vi "BCU参数读取-Auto.vi"(8 "CAN端口":u16(ring), 9 "设备索引号":u16(ring), 10 "CAN卡类型":u32(ring)=21, 11 "Myindex":dbl=1.0) -> (3 "成功":bool)   [LabVIEW 2013] (continued)
                n4250 = local write "命令序号"(w6047) -> ()
                n4251 = local write "命令"(w6052) -> ()
                n4252 = local write "控制1"(TRUE ("控制1")) -> ()
                n4253 = local write "写?"(FALSE ("写?")) -> ()
                n4254 = local write "消除"(TRUE ("消除")) -> ()
                n4255 = global write "EV05全局变量1.vi" "流控帧 2"(TRUE ("流控帧 2")) -> ()
                n4256 = global write "EV05全局变量1.vi" "流控帧"(FALSE ("流控帧")) -> ()
              }
              frame #2 {
                n4257 = flat-sequence {
                  tunnel: [w6095] -> w6094
                  tunnel: w6094 -> [w6102]
                  frame #0 {
                    n4258 = while {
                      tunnel: [w6096] -> w6095
                      i -> [w6100]
                      stop <- w6097 stop-if-true
                      n4259 = local read "继电器超时处理"() -> (w6096:bool)
                      n4260 = Greater Or Equal?(x=w6100, y=20) -> (x >= y?=w6098:bool)
                      n4261 = Wait Until Next ms Multiple(millisecond multiple=u32 100 ("毫秒倍数")) -> ()  [unwired: 1 out]
                      n4262 = Or(x=w6096, y=w6098) -> (x .or. y?=w6097:bool)
                    }
                  }
                  frame #1 {
                    n4263 = case shown="假" w6102 {
                      frame False {
                        n4264 = local read "DO1"() -> (w6104:bool)
                        n4265 = Not(x=w6104) -> (.not. x?=w6103:bool)
                        n4266 = local write "DO1"(w6103) -> ()
                        n4267 = One Button Dialog(message="DO控制处理超时" ("消息"), button name ("OK")="是" ("按钮名称（“确定”）")) -> ()  [unwired: 1 out]
                      }
                      frame True {
                      }
                    }
                  }
                }
              }
            }
          }
          event "DO2": Value Change {
            n4268 = event-data() -> ("NewVal"=w6107:bool)  [unwired: 6 out]
            n4269 = stacked-sequence {
              tunnel: w6107 -> [_ w6120 _]
              frame #0 {
                w6110 = FALSE ("清BUFF")
                n4270 = local write "继电器超时处理"(FALSE ("继电器超时处理")) -> ()
                n4271 = local write "主从选择"(enum32{"主板", "从板"}."主板" ("主从选择")) -> ()
                n4272 = local write "清BUFF"(w6110) -> ()
                n4273 = local write "正级继电器 10"(w6110) -> ()
              }
              frame #1 {
                n4274 = case shown="真" w6120 {
                  selector: w6120 -> [w6135 w6155]
                  tunnel: [w6134 w6154] -> w6119
                  tunnel: [w6122 w6142] -> w6114
                  frame False {
                    w6130 = 256.0 ("y")
                    w6122 = u32 2 ("命令序号")
                    w6134 = u8 192 ("命令")
                    n4275 = local read "动作保持时间"() -> (w6131:dbl)
                    n4276 = Quotient & Remainder(x=w6131, y=w6130) -> (x-y*floor(x/y)=w6123:dbl, floor(x/y)=w6127:dbl)
                    n4277 = Quotient & Remainder(x=w6127, y=w6130) -> (x-y*floor(x/y)=w6124:dbl, floor(x/y)=w6128:dbl)
                    n4278 = Quotient & Remainder(x=w6128, y=w6130) -> (x-y*floor(x/y)=w6125:dbl, floor(x/y)=w6129:dbl)
                    n4279 = local read "设备索引号"() -> (w6139:u16)
                    n4280 = local read "CAN卡类型"() -> (w6140:u32)
                    n4281 = local read "CAN端口"() -> (w6138:u16)
                    n4282 = Boolean To (0,1)(Boolean=w6135) -> (0, 1=w6132:i16)
                    n4283 = Quotient & Remainder(x=w6129, y=w6130) -> (x-y*floor(x/y)=w6126:dbl)  [unwired: 1 out]
                    n4284 = Build Array(i16 2 ("元素"), w6132, w6126, w6125, w6124, w6123, 0.0 ("元素")) -> (w6136:dbl[])
                    n4285 = call "多帧发送机制(EV05).vi"("can卡类型"=w6140, "设备索引号"=w6139, "CAN端口"=w6138, "命令"=w6134, "板号"=u8 0, "命令序号"=w6122, "输入数据"=w6136) -> ()  [unwired: 2 in, 11 out]
                  }
                  frame True {
                    w6150 = 256.0 ("y")
                    w6142 = u32 2 ("命令序号")
                    w6154 = u8 192 ("命令")
                    n4286 = local read "动作保持时间"() -> (w6151:dbl)
                    n4287 = Quotient & Remainder(x=w6151, y=w6150) -> (x-y*floor(x/y)=w6143:dbl, floor(x/y)=w6147:dbl)
                    n4288 = Quotient & Remainder(x=w6147, y=w6150) -> (x-y*floor(x/y)=w6144:dbl, floor(x/y)=w6148:dbl)
                    n4289 = Quotient & Remainder(x=w6148, y=w6150) -> (x-y*floor(x/y)=w6145:dbl, floor(x/y)=w6149:dbl)
                    n4290 = local read "设备索引号"() -> (w6159:u16)
                    n4291 = local read "CAN卡类型"() -> (w6160:u32)
                    n4292 = local read "CAN端口"() -> (w6158:u16)
                    n4293 = Boolean To (0,1)(Boolean=w6155) -> (0, 1=w6152:i16)
                    n4294 = Quotient & Remainder(x=w6149, y=w6150) -> (x-y*floor(x/y)=w6146:dbl)  [unwired: 1 out]
                    n4295 = Build Array(i16 2 ("元素"), w6152, w6146, w6145, w6144, w6143, 0.0 ("元素")) -> (w6156:dbl[])
                    n4296 = call "多帧发送机制(EV05).vi"("can卡类型"=w6160, "设备索引号"=w6159, "CAN端口"=w6158, "命令"=w6154, "板号"=u8 0, "命令序号"=w6142, "输入数据"=w6156) -> ()  [unwired: 2 in, 11 out]
                  }
                }
                n4297 = local write "命令序号"(w6114) -> ()
                n4298 = local write "命令"(w6119) -> ()
                n4299 = local write "控制1"(TRUE ("控制1")) -> ()
                n4300 = local write "写?"(FALSE ("写?")) -> ()
                n4301 = local write "消除"(TRUE ("消除")) -> ()
                n4302 = global write "EV05全局变量1.vi" "流控帧 2"(TRUE ("流控帧 2")) -> ()
                n4303 = global write "EV05全局变量1.vi" "流控帧"(FALSE ("流控帧")) -> ()
              }
              frame #2 {
                n4304 = flat-sequence {
                  tunnel: [w6162] -> w6161
                  tunnel: w6161 -> [w6169]
                  frame #0 {
                    n4305 = while {
                      tunnel: [w6163] -> w6162
                      i -> [w6167]
                      stop <- w6164 stop-if-true
                      n4306 = local read "继电器超时处理"() -> (w6163:bool)
                      n4307 = Greater Or Equal?(x=w6167, y=20) -> (x >= y?=w6165:bool)
                      n4308 = Wait Until Next ms Multiple(millisecond multiple=u32 100 ("毫秒倍数")) -> ()  [unwired: 1 out]
                      n4309 = Or(x=w6163, y=w6165) -> (x .or. y?=w6164:bool)
                    }
                  }
                  frame #1 {
                    n4310 = case shown="假" w6169 {
                      frame False {
                        n4311 = local read "DO2"() -> (w6171:bool)
                        n4312 = Not(x=w6171) -> (.not. x?=w6170:bool)
                        n4313 = local write "DO2"(w6170) -> ()
                        n4314 = One Button Dialog(message="DO控制处理超时" ("消息"), button name ("OK")="是" ("按钮名称（“确定”）")) -> ()  [unwired: 1 out]
                      }
                      frame True {
                      }
                    }
                  }
                }
              }
            }
          }
          event "DO1 2": Value Change {
            n4315 = event-data() -> ("NewVal"=w6174:bool)  [unwired: 6 out]
            n4316 = stacked-sequence {
              tunnel: w6174 -> [_ w6188 _]
              frame #0 {
                w6177 = FALSE ("继电器超时处理")
                n4317 = local write "继电器超时处理"(w6177) -> ()
                n4318 = local write "正级继电器 11"(w6177) -> ()
                n4319 = local write "主从选择"(enum32{"主板", "从板"}."从板" ("主从选择")) -> ()
              }
              frame #1 {
                n4320 = case shown="假" w6188 {
                  selector: w6188 -> [w6203 w6223]
                  tunnel: [w6202 w6222] -> w6187
                  tunnel: [w6201 w6221] -> w6181
                  tunnel: [w6190 w6210] -> w6182
                  frame True {
                    w6198 = 256.0 ("y")
                    w6190 = u32 2 ("命令序号")
                    w6202 = u8 192 ("命令")
                    n4321 = local read "动作保持时间"() -> (w6199:dbl)
                    n4322 = Quotient & Remainder(x=w6199, y=w6198) -> (x-y*floor(x/y)=w6191:dbl, floor(x/y)=w6195:dbl)
                    n4323 = Quotient & Remainder(x=w6195, y=w6198) -> (x-y*floor(x/y)=w6192:dbl, floor(x/y)=w6196:dbl)
                    n4324 = Quotient & Remainder(x=w6196, y=w6198) -> (x-y*floor(x/y)=w6193:dbl, floor(x/y)=w6197:dbl)
                    n4325 = Quotient & Remainder(x=w6197, y=w6198) -> (x-y*floor(x/y)=w6194:dbl)  [unwired: 1 out]
                    n4326 = Boolean To (0,1)(Boolean=w6203) -> (0, 1=w6200:i16)
                    n4327 = local read "设备索引号"() -> (w6207:u16)
                    n4328 = local read "CAN卡类型"() -> (w6208:u32)
                    n4329 = local read "从板板号"() -> (w6201:u8)
                    n4330 = local read "CAN端口"() -> (w6206:u16)
                    n4331 = Build Array(i16 3 ("元素"), w6200, w6194, w6193, w6192, w6191, 0.0 ("元素")) -> (w6205:dbl[])
                    n4332 = call "多帧发送机制(EV05).vi"("can卡类型"=w6208, "设备索引号"=w6207, "CAN端口"=w6206, "命令"=w6202, "板号"=w6201, "命令序号"=w6190, "输入数据"=w6205) -> ()  [unwired: 2 in, 11 out]
                  }
                  frame False {
                    w6218 = 256.0 ("y")
                    w6210 = u32 2 ("命令序号")
                    w6222 = u8 192 ("命令")
                    n4333 = local read "动作保持时间"() -> (w6219:dbl)
                    n4334 = Quotient & Remainder(x=w6219, y=w6218) -> (x-y*floor(x/y)=w6211:dbl, floor(x/y)=w6215:dbl)
                    n4335 = Quotient & Remainder(x=w6215, y=w6218) -> (x-y*floor(x/y)=w6212:dbl, floor(x/y)=w6216:dbl)
                    n4336 = Quotient & Remainder(x=w6216, y=w6218) -> (x-y*floor(x/y)=w6213:dbl, floor(x/y)=w6217:dbl)
                    n4337 = Quotient & Remainder(x=w6217, y=w6218) -> (x-y*floor(x/y)=w6214:dbl)  [unwired: 1 out]
                    n4338 = Boolean To (0,1)(Boolean=w6223) -> (0, 1=w6220:i16)
                    n4339 = local read "设备索引号"() -> (w6227:u16)
                    n4340 = local read "CAN卡类型"() -> (w6228:u32)
                    n4341 = local read "从板板号"() -> (w6221:u8)
                    n4342 = local read "CAN端口"() -> (w6226:u16)
                    n4343 = Build Array(i16 1 ("元素"), w6220, w6214, w6213, w6212, w6211, 0.0 ("元素")) -> (w6225:dbl[])
                    n4344 = call "多帧发送机制(EV05).vi"("can卡类型"=w6228, "设备索引号"=w6227, "CAN端口"=w6226, "命令"=w6222, "板号"=w6221, "命令序号"=w6210, "输入数据"=w6225) -> ()  [unwired: 2 in, 11 out]
                  }
                }
                n4345 = local write "从板板号"(w6181) -> ()
                n4346 = local write "命令序号"(w6182) -> ()
                n4347 = local write "命令"(w6187) -> ()
                n4348 = local write "清BUFF"(FALSE ("清BUFF")) -> ()
                n4349 = local write "写?"(FALSE ("写?")) -> ()
                n4350 = local write "控制1"(TRUE ("控制1")) -> ()
                n4351 = global write "EV05全局变量1.vi" "流控帧"(FALSE ("流控帧")) -> ()
                n4352 = global write "EV05全局变量1.vi" "流控帧 2"(TRUE ("流控帧 2")) -> ()
                n4353 = local write "消除"(TRUE ("消除")) -> ()
              }
              frame #2 {
                n4354 = flat-sequence {
                  tunnel: [w6230] -> w6229
                  tunnel: w6229 -> [w6237]
                  frame #0 {
                    n4355 = while {
                      tunnel: [w6231] -> w6230
                      i -> [w6235]
                      stop <- w6232 stop-if-true
                      n4356 = local read "继电器超时处理"() -> (w6231:bool)
                      n4357 = Greater Or Equal?(x=w6235, y=20) -> (x >= y?=w6233:bool)
                      n4358 = Wait Until Next ms Multiple(millisecond multiple=u32 100 ("毫秒倍数")) -> ()  [unwired: 1 out]
                      n4359 = Or(x=w6231, y=w6233) -> (x .or. y?=w6232:bool)
                    }
                  }
                  frame #1 {
                    n4360 = case shown="假" w6237 {
                      frame False {
                        n4361 = local read "DO1 2"() -> (w6239:bool)
                        n4362 = Not(x=w6239) -> (.not. x?=w6238:bool)
                        n4363 = local write "DO1 2"(w6238) -> ()
                        n4364 = One Button Dialog(message="DO控制处理超时" ("消息"), button name ("OK")="是" ("按钮名称（“确定”）")) -> ()  [unwired: 1 out]
                      }
                      frame True {
                      }
                    }
                  }
                }
              }
            }
          }
          event "读取转换为写入": Value Change {
            n4365 = event-data() -> ("NewVal"=w6242:bool)  [unwired: 6 out]
            n4366 = case shown="真" w6242 {
              tunnel: w6246 -> [w6248 w6253]
              tunnel: [w6248 w6252] -> w6245
              tunnel: w6244 -> [w6247 w6251]
              tunnel: [w6247 w6250] -> w6243
              frame False {
              }
              frame True {
                n4367 = Enqueue Element(queue=w6253, element="读取转换为写入", error in (no error)=w6251) -> (queue out=w6252:refnum<queue>, error out=w6250:errorcluster)  [unwired: 2 out]
              }
            }
          }
          event "读取故障详细状态": Value Change {
            n4368 = event-data() -> ("NewVal"=w6258:bool)  [unwired: 5 out]
            n4369 = case shown="真" w6258 {
              tunnel: w6257 -> [w6260 w6273]
              tunnel: w6256 -> [w6259 w6272]
              tunnel: [w6260 w6271] -> w6255
              tunnel: [w6259 w6270] -> w6254
              frame False {
              }
              frame True {
                n4370 = disable-structure shown="启用" {
                  disable-tunnel: [w6282 TRUE ("发送成功")] -> w6269
                  frame Disabled {
                    n4371 = local read "主从选择"() -> (w6274:enum32{"主板", "从板"})
                    n4372 = case shown="\"主板\", 默认" w6274 {
                      tunnel: [0.0 ("FUNC") w6284] -> w6279
                      frame "主板", Default {
                      }
                      frame "从板" {
                        n4373 = local read "从板号"() -> (w6284:u8)
                      }
                    }
                    n4374 = local read "设备索引号"() -> (w6276:u16)
                    n4375 = local read "CAN卡类型"() -> (w6277:u32)
                    n4376 = local read "CAN端口"() -> (w6275:u16)
                    n4377 = call "标定授权发送.vi"("CAN卡类型"=w6277, "解锁类型"=enum16{"读取", "写", "下载"}."写", "设备索引号"=w6276, "CAN端口"=w6275, "是否连接"=TRUE, "板选择"=0, "FUNC"=w6279) -> ("发送成功"=w6282:bool)  [unwired: 8 out]
                  }
                  frame Enabled {
                  }
                }
                n4378 = case shown="真" w6269 {
                  tunnel: w6273 -> [w6287 w6292]
                  tunnel: w6272 -> [w6286 w6291]
                  tunnel: [w6287 w6289] -> w6271
                  tunnel: [w6286 w6288] -> w6270
                  frame False {
                  }
                  frame True {
                    n4379 = Enqueue Element(queue=w6292, element="读取故障状态" ("元素"), error in (no error)=w6291) -> (queue out=w6289:refnum<queue>, error out=w6288:errorcluster)  [unwired: 2 out]
                  }
                }
                n4380 = local write "电池故障"(string[][] []) -> ()
                n4381 = global write "EV05全局变量1.vi" "流控帧 2"(TRUE ("流控帧")) -> ()
                n4382 = local write "写?"(FALSE ("写?")) -> ()
                n4383 = local write "控制1"(TRUE ("控制1")) -> ()
                n4384 = local write "消除"(TRUE ("消除")) -> ()
                n4385 = local write "清BUFF"(FALSE ("清BUFF")) -> ()
                n4386 = global write "EV05全局变量1.vi" "流控帧"(FALSE ("流控帧")) -> ()
                n4387 = call <vilib>:"Set Busy.vi"("disable click? (T)"=FALSE) -> ()  [unwired: 3 in, 8 out]
              }
            }
          }
          event "项目软本读取": Value Change {
            n4388 = event-data() -> ("NewVal"=w6297:bool)  [unwired: 5 out]
            n4389 = case shown="真" w6297 {
              tunnel: w6296 -> [w6299 w6304]
              tunnel: w6295 -> [w6298 w6303]
              tunnel: [w6299 w6302] -> w6294
              tunnel: [w6298 w6301] -> w6293
              frame False {
              }
              frame True {
                n4390 = stacked-sequence {
                  tunnel: [w6307] -> _
                  frame #0 {
                    w6307 = FALSE ("disable click? (T)")
                    w6310 = FALSE ("写?")
                    n4391 = local write "写?"(w6310) -> ()
                    n4392 = global write "EV05全局变量1.vi" "写入超时"(w6310) -> ()
                    n4393 = local write "项目软件版本号"(" " ("项目软件版本号")) -> ()
                    n4394 = global write "EV05全局变量1.vi" "流控帧"(FALSE ("流控帧")) -> ()
                    n4395 = local write "主从选择"(enum32{"主板", "从板"}."主板" ("主从选择")) -> ()
                    n4396 = call <vilib>:"Set Busy.vi"("disable click? (T)"=w6307) -> ()  [unwired: 3 in, 8 out]
                    n4397 = local write "清BUFF"(FALSE ("清BUFF")) -> ()
                    n4398 = property on="保存版本信息" class="Bool (严格)"("Visible"=TRUE ("可见")) -> ()  [unwired: 2 in, 2 out]
                    n4399 = global write "EV05全局变量1.vi" "流控帧 2"(TRUE ("流控帧 2")) -> ()
                    n4400 = local write "控制1"(TRUE ("控制1")) -> ()
                    n4401 = local write "消除"(TRUE ("消除")) -> ()
                  }
                }
                n4402 = Enqueue Element(queue=w6304, element="项目软件版本读取" ("元素"), error in (no error)=w6303) -> (queue out=w6302:refnum<queue>, error out=w6301:errorcluster)  [unwired: 2 out]
              }
            }
          }
          event "读硬件版本号": Value Change {
            n4403 = event-data() -> ("NewVal"=w6319:bool)  [unwired: 5 out]
            n4404 = case shown="真" w6319 {
              tunnel: w6318 -> [w6321 w6328]
              tunnel: w6317 -> [w6320 w6327]
              tunnel: [w6321 w6326] -> w6316
              tunnel: [w6320 w6325] -> w6315
              frame False {
              }
              frame True {
                n4405 = global read "EV05全局变量1.vi" "授权功能"() -> (w6323:bool)
                n4406 = case shown="真" w6323 {
                  tunnel: [TRUE ("发送成功") w6347] -> w6324
                  frame False {
                  }
                  frame True {
                    n4407 = local read "设备索引号"() -> (w6342:u16)
                    n4408 = local read "CAN卡类型"() -> (w6343:u32)
                    n4409 = local read "CAN端口"() -> (w6341:u16)
                    n4410 = call "标定授权发送.vi"("CAN卡类型"=w6343, "解锁类型"=enum16{"读取", "写", "下载"}."读取", "设备索引号"=w6342, "CAN端口"=w6341, "是否连接"=TRUE, "板选择"=0, "FUNC"=u32 0) -> ("发送成功"=w6347:bool)  [unwired: 8 in]
                  }
                }
                n4411 = stacked-sequence {
                  tunnel: [w6331] -> w6322
                  frame #0 {
                    w6331 = TRUE ("控制1")
                    w6335 = FALSE ("写?")
                    n4412 = local write "写?"(w6335) -> ()
                    n4413 = global write "EV05全局变量1.vi" "写入超时"(w6335) -> ()
                    n4414 = call <vilib>:"Set Busy.vi"("disable click? (T)"=FALSE) -> ()  [unwired: 3 in, 8 out]
                    n4415 = local write "硬件版本号"("" ("硬件版本号")) -> ()
                    n4416 = property on="保存版本信息" class="Bool (严格)"("Visible"=TRUE ("可见")) -> ()  [unwired: 2 in, 2 out]
                    n4417 = local write "主从选择"(enum32{"主板", "从板"}."主板" ("主从选择")) -> ()
                    n4418 = local write "控制1"(w6331) -> ()
                    n4419 = local write "清BUFF"(FALSE ("清BUFF")) -> ()
                    n4420 = global write "EV05全局变量1.vi" "流控帧 2"(TRUE ("流控帧 2")) -> ()
                    n4421 = local write "消除"(TRUE ("消除")) -> ()
                    n4422 = global write "EV05全局变量1.vi" "流控帧"(FALSE ("流控帧")) -> ()
                  }
                }
                n4423 = case shown="真" w6324 {
                  tunnel: w6328 -> [w6349 w6354]
                  tunnel: w6327 -> [w6348 w6353]
                  tunnel: [w6349 w6351] -> w6326
                  tunnel: [w6348 w6350] -> w6325
                  tunnel: w6322 -> [_ _]
                  frame False {
                  }
                  frame True {
                    n4424 = Enqueue Element(queue=w6354, element="硬件版本读取" ("元素"), error in (no error)=w6353) -> (queue out=w6351:refnum<queue>, error out=w6350:errorcluster)  [unwired: 2 out]
                  }
                }
              }
            }
          }
          event "平台软件版本读取": Value Change {
            n4425 = event-data() -> ("NewVal"=w6359:bool)  [unwired: 5 out]
            n4426 = case shown="真" w6359 {
              tunnel: w6358 -> [w6361 w6366]
              tunnel: w6357 -> [w6360 w6365]
              tunnel: [w6361 w6364] -> w6356
              tunnel: [w6360 w6363] -> w6355
              frame False {
              }
              frame True {
                n4427 = stacked-sequence {
                  tunnel: [w6369] -> _
                  frame #0 {
                    w6369 = TRUE ("控制1")
                    w6373 = FALSE ("写?")
                    n4428 = call <vilib>:"Set Busy.vi"("disable click? (T)"=FALSE) -> ()  [unwired: 3 in, 8 out]
                    n4429 = local write "写?"(w6373) -> ()
                    n4430 = global write "EV05全局变量1.vi" "写入超时"(w6373) -> ()
                    n4431 = local write "平台软件版本号"(" " ("平台软件版本号")) -> ()
                    n4432 = local write "控制1"(w6369) -> ()
                    n4433 = local write "消除"(TRUE ("消除")) -> ()
                    n4434 = property on="保存版本信息" class="Bool (严格)"("Visible"=TRUE ("可见")) -> ()  [unwired: 2 in, 2 out]
                    n4435 = global write "EV05全局变量1.vi" "流控帧 2"(TRUE ("流控帧 2")) -> ()
                    n4436 = local write "主从选择"(enum32{"主板", "从板"}."主板" ("主从选择")) -> ()
                    n4437 = local write "清BUFF"(FALSE ("清BUFF")) -> ()
                    n4438 = global write "EV05全局变量1.vi" "流控帧"(FALSE ("流控帧")) -> ()
                  }
                }
                n4439 = Enqueue Element(queue=w6366, element="平台软件版本读取" ("元素"), error in (no error)=w6365) -> (queue out=w6364:refnum<queue>, error out=w6363:errorcluster)  [unwired: 2 out]
              }
            }
          }
          event "模块版本读取": Value Change {
            n4440 = event-data() -> ("NewVal"=w6381:bool)  [unwired: 5 out]
            n4441 = case shown="真" w6381 {
              tunnel: w6380 -> [w6383 w6390]
              tunnel: w6379 -> [w6382 w6389]
              tunnel: [w6383 w6388] -> w6378
              tunnel: [w6382 w6387] -> w6377
              frame False {
              }
              frame True {
                n4442 = global read "EV05全局变量1.vi" "授权功能"() -> (w6385:bool)
                n4443 = case shown="假" w6385 {
                  tunnel: [TRUE ("发送成功") w6408] -> w6386
                  frame False {
                  }
                  frame True {
                    n4444 = local read "设备索引号"() -> (w6403:u16)
                    n4445 = local read "CAN卡类型"() -> (w6404:u32)
                    n4446 = local read "CAN端口"() -> (w6402:u16)
                    n4447 = call "标定授权发送.vi"("CAN卡类型"=w6404, "解锁类型"=enum16{"读取", "写", "下载"}."读取", "设备索引号"=w6403, "CAN端口"=w6402, "是否连接"=TRUE, "板选择"=0, "FUNC"=u32 0) -> ("发送成功"=w6408:bool)  [unwired: 8 out]
                  }
                }
                n4448 = stacked-sequence {
                  tunnel: [w6393] -> w6384
                  frame #0 {
                    w6393 = TRUE ("控制1")
                    w6396 = FALSE ("写?")
                    n4449 = call <vilib>:"Set Busy.vi"("disable click? (T)"=FALSE) -> ()  [unwired: 3 in, 8 out]
                    n4450 = local write "写?"(w6396) -> ()
                    n4451 = global write "EV05全局变量1.vi" "写入超时"(w6396) -> ()
                    n4452 = local write "主从选择"(enum32{"主板", "从板"}."主板" ("主从选择")) -> ()
                    n4453 = local write "清BUFF"(FALSE ("清BUFF")) -> ()
                    n4454 = property on="保存版本信息" class="Bool (严格)"("Visible"=TRUE ("可见")) -> ()  [unwired: 2 in, 2 out]
                    n4455 = global write "EV05全局变量1.vi" "流控帧 2"(TRUE ("流控帧 2")) -> ()
                    n4456 = local write "控制1"(w6393) -> ()
                    n4457 = local write "消除"(TRUE ("消除")) -> ()
                    n4458 = global write "EV05全局变量1.vi" "流控帧"(FALSE ("流控帧")) -> ()
                  }
                }
                n4459 = case shown="真" w6386 {
                  tunnel: w6390 -> [w6410 w6415]
                  tunnel: w6389 -> [w6409 w6414]
                  tunnel: [w6410 w6412] -> w6388
                  tunnel: [w6409 w6411] -> w6387
                  tunnel: w6384 -> [_ _]
                  frame False {
                  }
                  frame True {
                    n4460 = Enqueue Element(queue=w6415, element="模块软件版本读取" ("元素"), error in (no error)=w6414) -> (queue out=w6412:refnum<queue>, error out=w6411:errorcluster)  [unwired: 2 out]
                  }
                }
              }
            }
          }
          event "保存版本信息": Value Change {
            n4461 = event-data() -> ("NewVal"=w6416:bool)  [unwired: 6 out]
            n4462 = case shown="真" w6416 {
              frame False {
              }
              frame True {
                n4463 = stacked-sequence {
                  seq-local: [w6420 _] -> [_ w6422]
                  seq-local: [w6419 _] -> [_ w6421]
                  frame #0 {
                    n4464 = call "请输入从板个数"() -> ("从板个数"=w6420:dbl, "确定"=w6419:bool)  [unwired: 17 in, 1 out]
                  }
                  frame #1 {
                    n4465 = case shown="真" w6421 {
                      tunnel: w6422 -> [_ w6425]
                      frame False {
                      }
                      frame True {
                        n4466 = call <vilib>:"Application Directory.vi"() -> ("Application Directory"=w6437:path)
                        n4467 = Build Path(base path=w6437, name or relative path="SaveData" ("名称或相对路径")) -> (appended path=w6435:path)
                        n4468 = local read "模块版本名称"() -> (w6430:string[][])
                        n4469 = local read "项目软件版本"() -> (w6427:string[])
                        n4470 = local read "模块版本值"() -> (w6429:string[][])
                        n4471 = local read "平台软件版本"() -> (w6426:string[])
                        n4472 = local read "模块个数"() -> (w6423:u8[])
                        n4473 = local read "硬件版本"() -> (w6428:string[])
                        n4474 = call "文件对话框3"("start path"=w6435, "prompt"="选择要保存数据的位置", "default name"="BMS版本信息.txt") -> ("selected path"=w6431:path, "cancelled"=w6432:bool)  [unwired: 9 in, 2 out]
                        n4475 = Increment(x=w6425) -> (x+1=w6424:dbl)
                        n4476 = for {
                          N: w6424 -> [_]
                          tunnel: w6432 -> [w6453]
                          tunnel: w6431 -> [w6452]
                          tunnel: w6430 -> [w6442] mode=indexing
                          tunnel: w6429 -> [w6440] mode=indexing
                          tunnel: w6428 -> [w6447] mode=indexing
                          tunnel: w6427 -> [w6446] mode=indexing
                          tunnel: w6426 -> [w6445] mode=indexing
                          tunnel: w6423 -> [w6438] mode=indexing
                          i -> [w6444]
                          w6450 = ""
                          w6457 = 0 ("索引")
                          n4477 = case shown="0, 默认" w6444 {
                            selector: w6444 -> [_ w6471]
                            tunnel: ["主板版本信息" w6472] -> w6462
                            tunnel: [FALSE TRUE] -> w6448
                            frame 0, Default {
                            }
                            frame 1.. {
                              n4478 = Number To Decimal String(number=w6471) -> (decimal integer string=w6470:string)  [unwired: 1 in]
                              n4479 = Concatenate Strings("从板", w6470, "版本信息") -> (w6472:string)
                            }
                          }
                          n4480 = Increment(x=w6438) -> (x+1=w6439:u8)
                          n4481 = Array Subset(array=w6442, length=w6439) -> (w6443:string[])  [unwired: 1 in]
                          n4482 = Array Subset(array=w6440, length=w6439) -> (w6441:string[])  [unwired: 1 in]
                          n4483 = Build Array(w6450, w6445, w6446, w6447, w6450) -> (w6456:string[])
                          n4484 = Build Array(w6462, "平台软件版本号", "项目软件版本号", "硬件版本号", "模块版本号") -> (w6458:string[])
                          n4485 = Insert Into Array(array=w6443, index=w6457, new element=w6458) -> (w6455:string[])
                          n4486 = Insert Into Array(array=w6441, index=w6457, new element=w6456) -> (w6454:string[])
                          n4487 = Build Array(w6455, w6454) -> (w6451:string[][])
                          n4488 = case shown="假" w6453 {
                            tunnel: w6452 -> [w6466 _]
                            tunnel: w6451 -> [w6465 _]
                            tunnel: w6448 -> [w6463 _]
                            frame False {
                              n4489 = call-poly <vilib>:"Write To Spreadsheet File.vi"("transpose? (no:F)"=TRUE, "append to file? (new file:F)"=w6463, "2D data"=w6465, "file path (dialog if empty)"=w6466) -> ()  [unwired: 4 in, 1 out]
                            }
                            frame True {
                            }
                          }
                        }
                      }
                    }
                  }
                }
              }
            }
          }
          event "单个写入": Value Change {
            n4490 = event-data() -> ("NewVal"=w6479:bool)  [unwired: 5 out]
            n4491 = case shown="真" w6479 {
              tunnel: w6478 -> [w6481 w6488]
              tunnel: w6477 -> [w6480 w6487]
              tunnel: [w6481 w6486] -> w6476
              tunnel: [w6480 w6485] -> w6475
              frame False {
              }
              frame True {
                w6483 = FALSE ("流控帧")
                w6482 = TRUE ("流控帧 2")
                n4492 = disable-structure shown="禁用" {
                  disable-tunnel: [w6497 TRUE ("发送成功")] -> w6484
                  frame Disabled {
                    n4493 = local read "主从选择"() -> (w6489:enum32{"主板", "从板"})
                    n4494 = case shown="\"主板\", 默认" w6489 {
                      tunnel: [0.0 ("FUNC") w6499] -> w6494
                      frame "主板", Default {
                      }
                      frame "从板" {
                        n4495 = local read "从板号"() -> (w6499:u8)
                      }
                    }
                    n4496 = local read "设备索引号"() -> (w6491:u16)
                    n4497 = local read "CAN卡类型"() -> (w6492:u32)
                    n4498 = local read "CAN端口"() -> (w6490:u16)
                    n4499 = call "标定授权发送.vi"("CAN卡类型"=w6492, "解锁类型"=enum16{"读取", "写", "下载"}."写", "设备索引号"=w6491, "CAN端口"=w6490, "是否连接"=TRUE, "板选择"=0, "FUNC"=w6494) -> ("发送成功"=w6497:bool)  [unwired: 8 out]
                  }
                  frame Enabled {
                  }
                }
                n4500 = case shown="真" w6484 {
                  tunnel: w6488 -> [w6502 w6506]
                  tunnel: w6487 -> [w6501 w6505]
                  tunnel: [w6502 w6508] -> w6486
                  tunnel: [w6501 w6507] -> w6485
                  frame False {
                  }
                  frame True {
                    n4501 = Flush Queue(queue=w6506, error in (no error)=w6505) -> (queue out=w6504:refnum<queue>, error out=w6503:errorcluster)  [unwired: 1 out]
                    n4502 = Enqueue Element(queue=w6504, element="单个写入" ("元素"), error in (no error)=w6503) -> (queue out=w6508:refnum<queue>, error out=w6507:errorcluster)  [unwired: 2 out]
                  }
                }
                n4503 = global write "EV05全局变量1.vi" "读取超时"(w6483) -> ()
                n4504 = global write "EV05全局变量1.vi" "流控帧"(w6483) -> ()
                n4505 = local write "消除"(w6482) -> ()
                n4506 = local write "控制1"(w6482) -> ()
                n4507 = global write "EV05全局变量1.vi" "流控帧 2"(w6482) -> ()
                n4508 = local write "写?"(w6482) -> ()
              }
            }
          }
          event "全部写入": Value Change {
            n4509 = event-data() -> ("NewVal"=w6514:bool)  [unwired: 5 out]
            n4510 = case shown="真" w6514 {
              tunnel: w6513 -> [w6516 w6524]
              tunnel: w6512 -> [w6515 w6523]
              tunnel: [w6516 w6522] -> w6511
              tunnel: [w6515 w6521] -> w6510
              frame False {
              }
              frame True {
                w6518 = FALSE ("流控帧")
                w6517 = TRUE ("流控帧 2")
                n4511 = global read "EV05全局变量1.vi" "授权功能"() -> (w6519:bool)
                n4512 = case shown="真" w6519 {
                  tunnel: [TRUE ("发送成功") w6534] -> w6520
                  frame False {
                  }
                  frame True {
                    n4513 = local read "主从选择"() -> (w6526:enum32{"主板", "从板"})
                    n4514 = case shown="\"从板\"" w6526 {
                      tunnel: [0.0 ("FUNC") w6536] -> w6527
                      frame "主板", Default {
                      }
                      frame "从板" {
                        n4515 = local read "从板号"() -> (w6536:u8)
                      }
                    }
                    n4516 = local read "设备索引号"() -> (w6529:u16)
                    n4517 = local read "CAN卡类型"() -> (w6530:u32)
                    n4518 = local read "CAN端口"() -> (w6528:u16)
                    n4519 = call "标定授权发送.vi"("CAN卡类型"=w6530, "解锁类型"=enum16{"读取", "写", "下载"}."写", "设备索引号"=w6529, "CAN端口"=w6528, "是否连接"=TRUE, "板选择"=0, "FUNC"=w6527) -> ("发送成功"=w6534:bool)  [unwired: 8 out]
                  }
                }
                n4520 = case shown="真" w6520 {
                  tunnel: w6524 -> [w6538 w6542]
                  tunnel: w6523 -> [w6537 w6541]
                  tunnel: [w6538 w6544] -> w6522
                  tunnel: [w6537 w6543] -> w6521
                  frame False {
                  }
                  frame True {
                    n4521 = Flush Queue(queue=w6542, error in (no error)=w6541) -> (queue out=w6540:refnum<queue>, error out=w6539:errorcluster)  [unwired: 1 out]
                    n4522 = Enqueue Element(queue=w6540, element="全部写入" ("元素"), error in (no error)=w6539) -> (queue out=w6544:refnum<queue>, error out=w6543:errorcluster)  [unwired: 1 in, 1 out]
                  }
                }
                n4523 = global write "EV05全局变量1.vi" "读取超时"(w6518) -> ()
                n4524 = global write "EV05全局变量1.vi" "流控帧"(w6518) -> ()
                n4525 = local write "消除"(w6517) -> ()
                n4526 = local write "控制1"(w6517) -> ()
                n4527 = global write "EV05全局变量1.vi" "流控帧 2"(w6517) -> ()
                n4528 = local write "写?"(w6517) -> ()
              }
            }
          }
          event "单个读取": Value Change {
            n4529 = event-data() -> ("NewVal"=w6550:bool)  [unwired: 5 out]
            n4530 = case shown="真" w6550 {
              tunnel: w6549 -> [w6552 w6560]
              tunnel: w6548 -> [w6551 w6559]
              tunnel: [w6552 w6558] -> w6547
              tunnel: [w6551 w6557] -> w6546
              frame False {
              }
              frame True {
                w6553 = FALSE ("流控帧")
                w6554 = TRUE ("流控帧 2")
                n4531 = global read "EV05全局变量1.vi" "授权功能"() -> (w6555:bool)
                n4532 = case shown="假" w6555 {
                  tunnel: [TRUE ("发送成功") w6569] -> w6556
                  frame False {
                  }
                  frame True {
                    n4533 = local read "设备索引号"() -> (w6563:u16)
                    n4534 = local read "CAN卡类型"() -> (w6564:u32)
                    n4535 = local read "CAN端口"() -> (w6562:u16)
                    n4536 = call "标定授权发送.vi"("CAN卡类型"=w6564, "解锁类型"=enum16{"读取", "写", "下载"}."读取", "设备索引号"=w6563, "CAN端口"=w6562, "是否连接"=TRUE, "板选择"=0, "FUNC"=u32 1) -> ("发送成功"=w6569:bool)  [unwired: 8 out]
                  }
                }
                n4537 = case shown="真" w6556 {
                  tunnel: w6560 -> [w6571 w6575]
                  tunnel: w6559 -> [w6570 w6573]
                  tunnel: [w6571 w6577] -> w6558
                  tunnel: [w6570 w6576] -> w6557
                  frame False {
                  }
                  frame True {
                    n4538 = Flush Queue(queue=w6575, error in (no error)=w6573) -> (queue out=w6574:refnum<queue>, error out=w6572:errorcluster)  [unwired: 1 out]
                    n4539 = Enqueue Element(queue=w6574, element="单个读取" ("元素"), error in (no error)=w6572) -> (queue out=w6577:refnum<queue>, error out=w6576:errorcluster)  [unwired: 2 out]
                  }
                }
                n4540 = global write "EV05全局变量1.vi" "写入超时"(w6553) -> ()
                n4541 = global write "EV05全局变量1.vi" "流控帧"(w6553) -> ()
                n4542 = local write "写?"(w6553) -> ()
                n4543 = local write "消除"(w6554) -> ()
                n4544 = local write "控制1"(w6554) -> ()
                n4545 = global write "EV05全局变量1.vi" "流控帧 2"(w6554) -> ()
              }
            }
          }
          event "全部读取": Value Change {
            n4546 = event-data() -> ("NewVal"=w6583:bool)  [unwired: 5 out]
            n4547 = case shown="真" w6583 {
              tunnel: w6582 -> [w6585 w6589]
              tunnel: w6581 -> [w6584 w6588]
              tunnel: [w6585 w6587] -> w6580
              tunnel: [w6584 w6586] -> w6579
              frame False {
              }
              frame True {
                n4548 = stacked-sequence {
                  seq-local: [w6594 _] -> [_ _]
                  seq-local: [w6593 _] -> [_ _]
                  tunnel: w6589 -> [w6596 w6625]
                  tunnel: w6588 -> [w6595 w6624]
                  tunnel: [_ w6629] -> w6587
                  tunnel: [_ w6628] -> w6586
                  frame #0 {
                    w6590 = FALSE ("布尔")
                    n4549 = local read "路径"() -> (w6592:path)
                    n4550 = Empty String/Path?(string/path=w6592) -> (empty?=w6591:bool)
                    n4551 = case shown="假" w6591 {
                      tunnel: w6596 -> [w6603 w6621]
                      tunnel: w6595 -> [w6602 w6620]
                      tunnel: [w6599 w6620] -> w6594
                      tunnel: [w6598 w6621] -> w6593
                      frame False {
                        n4552 = global read "EV05全局变量1.vi" "授权功能"() -> (w6600:bool)
                        n4553 = case shown="真" w6600 {
                          tunnel: [TRUE ("发送成功") w6612] -> w6601
                          frame False {
                          }
                          frame True {
                            n4554 = local read "设备索引号"() -> (w6606:u16)
                            n4555 = local read "CAN卡类型"() -> (w6607:u32)
                            n4556 = local read "CAN端口"() -> (w6605:u16)
                            n4557 = call "标定授权发送.vi"("CAN卡类型"=w6607, "解锁类型"=enum16{"读取", "写", "下载"}."读取", "设备索引号"=w6606, "CAN端口"=w6605, "是否连接"=TRUE, "板选择"=0, "FUNC"=u32 1) -> ("发送成功"=w6612:bool)  [unwired: 8 out]
                          }
                        }
                        n4558 = case shown="真" w6601 {
                          tunnel: w6603 -> [w6614 w6619]
                          tunnel: w6602 -> [w6613 w6618]
                          tunnel: [w6614 w6616] -> w6598
                          tunnel: [w6613 w6615] -> w6599
                          frame False {
                          }
                          frame True {
                            n4559 = Enqueue Element(queue=w6619, element="读配置文件" ("元素"), error in (no error)=w6618) -> (queue out=w6616:refnum<queue>, error out=w6615:errorcluster)  [unwired: 2 out]
                          }
                        }
                        n4560 = Wait Until Next ms Multiple(millisecond multiple=u32 200 ("毫秒倍数")) -> ()  [unwired: 1 out]
                      }
                      frame True {
                      }
                    }
                    n4561 = local write "1 6"(w6590) -> ()
                    n4562 = local write "1 7"(w6590) -> ()
                    n4563 = local write "1 8"(w6590) -> ()
                    n4564 = local write "1 9"(w6590) -> ()
                    n4565 = local write "1 10"(w6590) -> ()
                    n4566 = local write "1 12"(w6590) -> ()
                  }
                  frame #1 {
                    w6622 = FALSE ("流控帧")
                    w6623 = TRUE ("流控帧 2")
                    n4567 = global read "EV05全局变量1.vi" "授权功能"() -> (w6626:bool)
                    n4568 = case shown="假" w6626 {
                      tunnel: [TRUE ("发送成功") w6638] -> w6627
                      frame False {
                      }
                      frame True {
                        n4569 = local read "设备索引号"() -> (w6632:u16)
                        n4570 = local read "CAN卡类型"() -> (w6633:u32)
                        n4571 = local read "CAN端口"() -> (w6631:u16)
                        n4572 = call "标定授权发送.vi"("CAN卡类型"=w6633, "解锁类型"=enum16{"读取", "写", "下载"}."读取", "设备索引号"=w6632, "CAN端口"=w6631, "是否连接"=TRUE, "板选择"=0, "FUNC"=u32 1) -> ("发送成功"=w6638:bool)  [unwired: 8 out]
                      }
                    }
                    n4573 = case shown="真" w6627 {
                      tunnel: w6625 -> [w6640 w6641]
                      tunnel: w6624 -> [w6639 w6644]
                      tunnel: [w6640 w6646] -> w6629
                      tunnel: [w6639 w6645] -> w6628
                      frame False {
                      }
                      frame True {
                        n4574 = Flush Queue(queue=w6641, error in (no error)=w6644) -> (queue out=w6642:refnum<queue>, error out=w6643:errorcluster)  [unwired: 1 out]
                        n4575 = Enqueue Element(queue=w6642, element="全部读取" ("元素"), error in (no error)=w6643) -> (queue out=w6646:refnum<queue>, error out=w6645:errorcluster)  [unwired: 2 out]
                      }
                    }
                    n4576 = global write "EV05全局变量1.vi" "写入超时"(w6622) -> ()
                    n4577 = global write "EV05全局变量1.vi" "流控帧"(w6622) -> ()
                    n4578 = local write "写?"(w6622) -> ()
                    n4579 = local write "消除"(w6623) -> ()
                    n4580 = local write "控制1"(w6623) -> ()
                    n4581 = global write "EV05全局变量1.vi" "流控帧 2"(w6623) -> ()
                  }
                }
              }
            }
          }
          event "开启均衡": Value Change {
            n4582 = event-data() -> ("NewVal"=w6652:bool)  [unwired: 5 out]
            n4583 = case shown="真" w6652 {
              tunnel: w6651 -> [w6654 w6661]
              tunnel: w6650 -> [w6653 w6660]
              tunnel: [w6654 w6659] -> w6649
              tunnel: [w6653 w6658] -> w6648
              frame False {
              }
              frame True {
                n4584 = global read "EV05全局变量1.vi" "授权功能"() -> (w6656:bool)
                n4585 = case shown="假" w6656 {
                  tunnel: [TRUE ("发送成功") w6671] -> w6657
                  frame False {
                  }
                  frame True {
                    n4586 = local read "主从选择"() -> (w6663:enum32{"主板", "从板"})
                    n4587 = case shown="\"从板\"" w6663 {
                      tunnel: [0.0 ("FUNC") w6673] -> w6664
                      frame "主板", Default {
                      }
                      frame "从板" {
                        n4588 = local read "从板号"() -> (w6673:u8)
                      }
                    }
                    n4589 = local read "设备索引号"() -> (w6666:u16)
                    n4590 = local read "CAN卡类型"() -> (w6667:u32)
                    n4591 = local read "CAN端口"() -> (w6665:u16)
                    n4592 = call "标定授权发送.vi"("CAN卡类型"=w6667, "解锁类型"=enum16{"读取", "写", "下载"}."写", "设备索引号"=w6666, "CAN端口"=w6665, "是否连接"=TRUE, "板选择"=0, "FUNC"=w6664) -> ("发送成功"=w6671:bool)  [unwired: 8 out]
                  }
                }
                n4593 = case shown="真" w6657 {
                  tunnel: w6661 -> [w6675 w6680]
                  tunnel: w6660 -> [w6674 w6679]
                  tunnel: [w6675 w6677] -> w6659
                  tunnel: [w6674 w6676] -> w6658
                  frame False {
                  }
                  frame True {
                    n4594 = Enqueue Element(queue=w6680, element="开启均衡" ("元素"), error in (no error)=w6679) -> (queue out=w6677:refnum<queue>, error out=w6676:errorcluster)  [unwired: 2 out]
                  }
                }
                n4595 = call <vilib>:"Set Busy.vi"("disable click? (T)"=TRUE) -> ()  [unwired: 3 in, 8 out]
              }
            }
          }
          event "关闭均衡": Value Change {
            n4596 = event-data() -> ("NewVal"=w6685:bool)  [unwired: 5 out]
            n4597 = case shown="真" w6685 {
              tunnel: w6684 -> [w6687 w6694]
              tunnel: w6683 -> [w6686 w6693]
              tunnel: [w6687 w6692] -> w6682
              tunnel: [w6686 w6691] -> w6681
              frame False {
              }
              frame True {
                n4598 = global read "EV05全局变量1.vi" "授权功能"() -> (w6689:bool)
                n4599 = case shown="假" w6689 {
                  tunnel: [TRUE ("发送成功") w6704] -> w6690
                  frame False {
                  }
                  frame True {
                    n4600 = local read "主从选择"() -> (w6696:enum32{"主板", "从板"})
                    n4601 = case shown="\"从板\"" w6696 {
                      tunnel: [0.0 ("FUNC") w6706] -> w6697
                      frame "主板", Default {
                      }
                      frame "从板" {
                        n4602 = local read "从板号"() -> (w6706:u8)
                      }
                    }
                    n4603 = local read "设备索引号"() -> (w6699:u16)
                    n4604 = local read "CAN卡类型"() -> (w6700:u32)
                    n4605 = local read "CAN端口"() -> (w6698:u16)
                    n4606 = call "标定授权发送.vi"("CAN卡类型"=w6700, "解锁类型"=enum16{"读取", "写", "下载"}."写", "设备索引号"=w6699, "CAN端口"=w6698, "是否连接"=TRUE, "板选择"=0, "FUNC"=w6697) -> ("发送成功"=w6704:bool)  [unwired: 8 out]
                  }
                }
                n4607 = case shown="真" w6690 {
                  tunnel: w6694 -> [w6708 w6713]
                  tunnel: w6693 -> [w6707 w6712]
                  tunnel: [w6708 w6710] -> w6692
                  tunnel: [w6707 w6709] -> w6691
                  frame False {
                  }
                  frame True {
                    n4608 = Enqueue Element(queue=w6713, element="关闭均衡" ("元素"), error in (no error)=w6712) -> (queue out=w6710:refnum<queue>, error out=w6709:errorcluster)  [unwired: 2 out]
                  }
                }
                n4609 = call <vilib>:"Set Busy.vi"("disable click? (T)"=TRUE) -> ()  [unwired: 3 in, 8 out]
              }
            }
          }
          event "强制开启均衡": Value Change {
            n4610 = event-data() -> ("NewVal"=w6718:bool)  [unwired: 5 out]
            n4611 = case shown="真" w6718 {
              tunnel: w6717 -> [w6720 w6727]
              tunnel: w6716 -> [w6719 w6726]
              tunnel: [w6720 w6725] -> w6715
              tunnel: [w6719 w6724] -> w6714
              frame False {
              }
              frame True {
                n4612 = global read "EV05全局变量1.vi" "授权功能"() -> (w6722:bool)
                n4613 = case shown="假" w6722 {
                  tunnel: [TRUE ("发送成功") w6737] -> w6723
                  frame False {
                  }
                  frame True {
                    n4614 = local read "主从选择"() -> (w6729:enum32{"主板", "从板"})
                    n4615 = case shown="\"从板\"" w6729 {
                      tunnel: [0.0 ("FUNC") w6739] -> w6730
                      frame "主板", Default {
                      }
                      frame "从板" {
                        n4616 = local read "从板号"() -> (w6739:u8)
                      }
                    }
                    n4617 = local read "设备索引号"() -> (w6732:u16)
                    n4618 = local read "CAN卡类型"() -> (w6733:u32)
                    n4619 = local read "CAN端口"() -> (w6731:u16)
                    n4620 = call "标定授权发送.vi"("CAN卡类型"=w6733, "解锁类型"=enum16{"读取", "写", "下载"}."写", "设备索引号"=w6732, "CAN端口"=w6731, "是否连接"=TRUE, "板选择"=0, "FUNC"=w6730) -> ("发送成功"=w6737:bool)  [unwired: 8 out]
                  }
                }
                n4621 = case shown="真" w6723 {
                  tunnel: w6727 -> [w6741 w6746]
                  tunnel: w6726 -> [w6740 w6745]
                  tunnel: [w6741 w6743] -> w6725
                  tunnel: [w6740 w6742] -> w6724
                  frame False {
                  }
                  frame True {
                    n4622 = Enqueue Element(queue=w6746, element="强制均衡" ("元素"), error in (no error)=w6745) -> (queue out=w6743:refnum<queue>, error out=w6742:errorcluster)  [unwired: 2 out]
                  }
                }
                n4623 = call <vilib>:"Set Busy.vi"("disable click? (T)"=TRUE) -> ()  [unwired: 3 in, 8 out]
              }
            }
          }
        }
        n4624 = Unbundle By Name(w3971) -> ("status"=w3970:bool)
        n4625 = Or(x=w3970, y=w3972) -> (x .or. y?=w3973:bool)
      }
      n4626 = Release Queue(queue=w3967, force destroy? (F)=TRUE ("强制销毁？(F)"), error in (no error)=w3966) -> (error out=w3964:errorcluster)  [unwired: 2 out]
      n4627 = call <vilib>:"Clear Errors.vi"("error in (no error)"=w3964) -> ()  [unwired: 7 out]
    }
    frame Enabled {
    }
  }
  n4628 = Release Queue(queue=w29, force destroy? (F)=TRUE ("强制销毁？(F)"), error in (no error)=w28) -> (error out=w31:errorcluster)  [unwired: 2 out]
  n4629 = call <vilib>:"Clear Errors.vi"("error in (no error)"=w31) -> ()  [unwired: 7 out]
  n4630 = local write "面板选择"(T7."读写参数" ("面板选择")) -> ()
